vi "IV programa 3_3.vi"() -> ()   [LabVIEW 2020]
panel:
  in  "B 2":dbl
  in  "A":dbl
  out "XY Graph":cluster{dbl[], dbl[]}(graph)
  out "theta":dbl[](array[numeric])
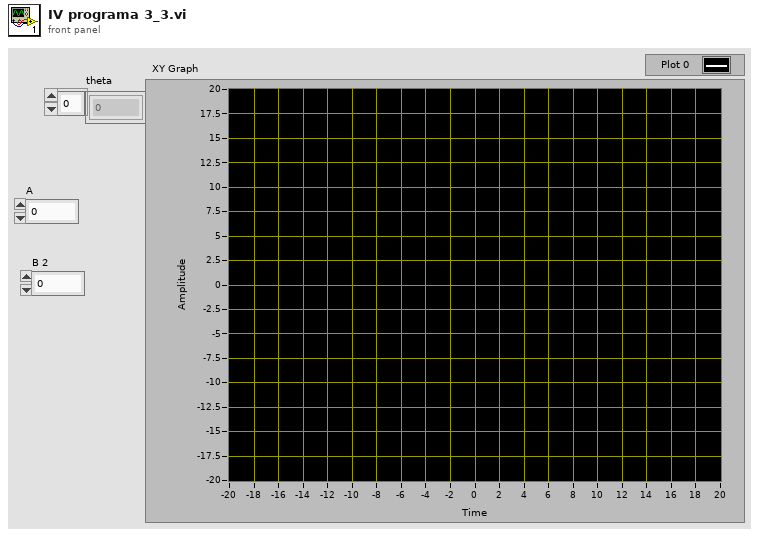
[diagram p1: front panel]
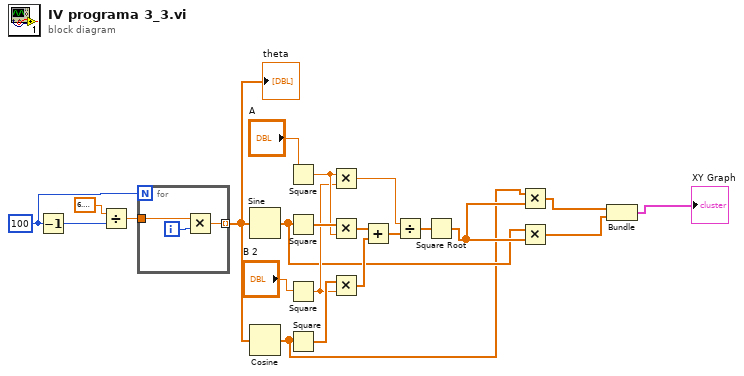
[diagram p0: block diagram]
diagram:
  w22 = 100
  n1 = Decrement(x=w22) -> (x-1=w20:i32)
  n2 = Divide(x=6.283185307179586, y=w20) -> (x/y=w19:dbl)
  n3 = for {
    N: w22 -> [_]
    tunnel: w19 -> [w24]
    tunnel: [w23] -> w18 mode=indexing
    i -> [w25]
    n4 = Multiply(x=w24, y=w25) -> (x*y=w23:dbl)
  }
  "theta" <- w18
  n5 = Sine(x=w18) -> (sin(x)=w7:dbl[])
  n6 = Cosine(x=w18) -> (cos(x)=w6:dbl[])
  n7 = Square(x="A") -> (x^2=w15:dbl)
  n8 = Square(x=w7) -> (x^2=w17:dbl[])
  n9 = Square(x="B 2") -> (x^2=w14:dbl)
  n10 = Square(x=w6) -> (x^2=w16:dbl[])
  n11 = Multiply(x=w15, y=w14) -> (x*y=w10:dbl)
  n12 = Multiply(x=w17, y=w15) -> (x*y=w13:dbl[])
  n13 = Multiply(x=w16, y=w14) -> (x*y=w12:dbl[])
  n14 = Add(x=w13, y=w12) -> (x+y=w11:dbl[])
  n15 = Divide(x=w10, y=w11) -> (x/y=w9:dbl[])
  n16 = Square Root(x=w9) -> (sqrt(x)=w8:dbl[])
  n17 = Multiply(x=w6, y=w8) -> (x*y=w5:dbl[])
  n18 = Multiply(x=w7, y=w8) -> (x*y=w4:dbl[])
  n19 = Bundle(w5, w4) -> (→"XY Graph":cluster{dbl[], dbl[]})  [unwired: 1 in]
